vi "rsidr_core_global.vi"() -> ()   [LabVIEW 2020, in "Rohde&Schwarz CMWXP NR FR1 Measurement.lvlib"] (continued)
i9, i10, i11, i12, i13, i14, i15, i16, i17, i18, i19, i20, i21, i22, i23, i24, i25, i26, i27, i28, i29, i30, i31, i32\r\n\nRemote-control command(s):\nCONFigure:NRSub:MEAS<i>:MEValuation:LIMit:QPSK:FERRor"}, {"Level"=5, "Class Only"=FALSE, "Identifier"="RSCMWXPNRFR1M_ATTR_MULTI_EVAL_MEAS_LIMIT_QPSK_IQ_OFFSET", "Descriptive Name"="Multi Eval Meas Limit QPSK IQ Offset", "Data Type"=enum."RawString", "Command"="CONF:NRS:MEAS{instance}:MEV:LIM:QPSK:IQOF", "Access"=enum."Read/Write", "Range Table"="", "Read Callback"="", "Write Callback"="", "Range Callback"="", "Check Callback"="", "Rngtable Callback"="", "Coerce Callback"="", "Supported Models"="", "Instrument Options"="", "Check Status Callback"="", "Flags"=0, "Help"="Defines upper limits for the I/Q origin offset (QPSK modulation). Four different I/Q origin offset limits can be set for four TX power ranges.\n\nSyntax:\nCONFigure:NRSub:MEAS<i>:MEValuation:LIMit:QPSK:IQOFfset <Enable>, <Offset0>, <Offset1>,<Offset2>,<Offset3>\n\n<Enable>\nValid Values:\nOFF: disables the limit check\nON: enables the limit check\n\n<Offset0>\nI/Q origin offset limit for TX power > 10 dBm\nnumeric\nValid Values: -256 dBc to 256 dBc\n\n<Offset1>\nI/Q origin offset limit for TX power > 0 dBm\nnumeric\nValid Values: -256 dBc to 256 dBc\n\n<Offset2>\nI/Q origin offset limit for TX power > -30 dBm\nnumeric\nValid Values: -256 dBc to 256 dBc\n\n<Offset3>\nI/Q origin offset limit for TX power > -40 dBm\nnumeric\nValid Values: -256 dBc to 256 dBc\n\nAvailable Repeated Capabilities:\ninstance: i0, i1, i2, i3, i4, i5, i6, i7, i8, i9, i10, i11, i12, i13, i14, i15, i16, i17, i18, i19, i20, i21, i22, i23, i24, i25, i26, i27, i28, i29, i30, i31, i32\r\n\nRemote-control command(s):\nCONFigure:NRSub:MEAS<i>:MEValuation:LIMit:QPSK:IQOFfset"}, {"Level"=5, "Class Only"=FALSE, "Identifier"="RSCMWXPNRFR1M_ATTR_MULTI_EVAL_MEAS_LIMIT_QPSK_INBAND_EMISSION", "Descriptive Name"="Multi Eval Meas Limit QPSK Inband Emission", "Data Type"=enum."RawString", "Command"="CONF:NRS:MEAS{instance}:MEV:LIM:QPSK:IBE", "Access"=enum."Read/Write", "Range Table"="", "Read Callback"="", "Write Callback"="", "Range Callback"="", "Check Callback"="", "Rngtable Callback"="", "Coerce Callback"="", "Supported Models"="", "Instrument Options"="", "Check Status Callback"="", "Flags"=0, "Help"="Defines parameters used for calculation of an upper limit for the inband emission (QPSK modulation), see 'Inband Emissions Limits'.\n\nSyntax:\nCONFigure:NRSub:MEAS<i>:MEValuation:LIMit:QPSK:IBE <Enable>, <Minimum>, <EVM>, <RBPower>, <IQImageLesser>, <IQImageGreater>\n\n<Enable>\nValid Values:\nOFF: disables the limit check\nON: enables the limit check\n\n<Minimum>\nnumeric\nValid Values: -256 dB to 256 dB\n\n<EVM>\nnumeric\nValid Values: 0 % to 100 %\n\n<RBPower>\nnumeric\nValid Values: -256 dBm to 256 dBm\n\n<IQImageLesser>\nIQ image for low TX power range\nnumeric\nValid Values: -256 dB to 256 dB\n \n<IQImageGreater>\nIQ image for high TX power range\nnumeric\nValid Values: -256 dB  to  256 dB\n\nAvailable Repeated Capabilities:\ninstance: i0, i1, i2, i3, i4, i5, i6, i7, i8, i9, i10, i11, i12, i13, i14, i15, i16, i17, i18, i19, i20, i21, i22, i23, i24, i25, i26, i27, i28, i29, i30, i31, i32\r\n\nRemote-control command(s):\nCONFigure:NRSub:MEAS<i>:MEValuation:LIMit:QPSK:IBE"}, {"Level"=5, "Class Only"=FALSE, "Identifier"="RSCMWXPNRFR1M_ATTR_MULTI_EVAL_MEAS_LIMIT_QPSK_INBAND_EMISSION_IQ_OFFSET", "Descriptive Name"="Multi Eval Meas Limit QPSK Inband Emission IQ Offset", "Data Type"=enum."RawString", "Command"="CONF:NRS:MEAS{instance}:MEV:LIM:QPSK:IBE:IQOF", "Access"=enum."Read/Write", "Range Table"="", "Read Callback"="", "Write Callback"="", "Range Callback"="", "Check Callback"="", "Rngtable Callback"="", "Coerce Callback"="", "Supported Models"="", "Instrument Options"="", "Check Status Callback"="", "Flags"=0, "Help"="Defines I/Q origin offset values used for calculation of an upper limit for the inband emission, for QPSK modulation. Four different values can be set for four TX power ranges.\n\nSyntax:\nCONFigure:NRSub:MEAS<i>:MEValuation:LIMit:QPSK:IBE:IQOFfset <Offset0>, <Offset1>,<Offset2>,<Offset3>\n\n<Offset0>\nI/Q origin offset limit for TX power > 10 dBm\nnumeric\nValid Values: -256 dBc to 256 dBc\n\n<Offset1>\nI/Q origin offset limit for TX power > 0 dBm\nnumeric\nValid Values: -256 dBc to 256 dBc\n\n<Offset2>\nI/Q origin offset limit for TX power > -30 dBm\nnumeric\nValid Values: -256 dBc to 256 dBc\n\n<Offset3>\nI/Q origin offset limit for TX power > -40 dBm\nnumeric\nValid Values: -256 dBc to 256 dBc\n\nAvailable Repeated Capabilities:\ninstance: i0, i1, i2, i3, i4, i5, i6, i7, i8, i9, i10, i11, i12, i13, i14, i15, i16, i17, i18, i19, i20, i21, i22, i23, i24, i25, i26, i27, i28, i29, i30, i31, i32\r\n\nRemote-control command(s):\nCONFigure:NRSub:MEAS<i>:MEValuation:LIMit:QPSK:IBE:IQOFfset"}, {"Level"=5, "Class Only"=FALSE, "Identifier"="RSCMWXPNRFR1M_ATTR_MULTI_EVAL_MEAS_LIMIT_QPSK_EQUALIZER_SPECTRUM_FLATNESS", "Descriptive Name"="Multi Eval Meas Limit QPSK Equalizer Spectrum Flatness", "Data Type"=enum."RawString", "Command"="CONF:NRS:MEAS{instance}:MEV:LIM:QPSK:ESFL", "Access"=enum."Read/Write", "Range Table"="", "Read Callback"="", "Write Callback"="", "Range Callback"="", "Check Callback"="", "Rngtable Callback"="", "Coerce Callback"="", "Supported Models"="", "Instrument Options"="", "Check Status Callback"="", "Flags"=0, "Help"="Defines limits for the equalizer spectrum flatness (QPSK modulation).\n\nSyntax:\nCONFigure:NRSub:MEAS<i>:MEValuation:LIMit:QPSK:ESFLatness <Enable>, <Range1>, <Range2>, <Max1Min2>, <Max2Min1>, <EdgeFrequency>\n\n<Enable>\nValid Values:\nOFF: disables the limit check\nON: enables the limit check\n\n<Range1>\nUpper limit for max(range 1) - min(range 1)\nnumeric\nValid Values: -256 dBpp to 256 dBpp \n\n<Range2>\nUpper limit for max(range 2) - min(range 2)\nnumeric\nValid Values: -256 dBpp to 256 dBpp \n\n<Max1Min2>\nUpper limit for max(range 1) - min(range 2)\nnumeric\nValid Values: -256 dB to 256 dB \n\n<Max2Min1>\nUpper limit for max(range 2) - min(range 1)\nnumeric\nValid Values: -256 dB to 256 dB\n\n<EdgeFrequency>\nBand edge distance of border between range 1 and range 2\nValid Values:\n0 MHz to 20 MHz\n\nAvailable Repeated Capabilities:\ninstance: i0, i1, i2, i3, i4, i5, i6, i7, i8, i9, i10, i11, i12, i13, i14, i15, i16, i17, i18, i19, i20, i21, i22, i23, i24, i25, i26, i27, i28, i29, i30, i31, i32\r\n\nRemote-control command(s):\nCONFigure:NRSub:MEAS<i>:MEValuation:LIMit:QPSK:ESFLatness"}, {"Level"=4, "Class Only"=TRUE, "Identifier"="", "Descriptive Name"="QAM", "Data Type"=enum."ViInt32", "Command"="", "Access"=enum."Read Only", "Range Table"="", "Read Callback"="", "Write Callback"="", "Range Callback"="", "Check Callback"="", "Rngtable Callback"="", "Coerce Callback"="", "Supported Models"="", "Instrument Options"="", "Check Status Callback"="", "Flags"=0, "Help"="16-QAM / 64-QAM / 256-QAM modulation  limits definition."}, {"Level"=5, "Class Only"=FALSE, "Identifier"="RSCMWXPNRFR1M_ATTR_MULTI_EVAL_MEAS_LIMIT_QAM_EVM", "Descriptive Name"="Multi Eval Meas Limit QAM EVM", "Data Type"=enum."RawString", "Command"="CONF:NRS:MEAS{instance}:MEV:LIM:QAM{QAM}:EVM", "Access"=enum."Read/Write", "Range Table"="", "Read Callback"="", "Write Callback"="", "Range Callback"="", "Check Callback"="", "Rngtable Callback"="", "Coerce Callback"="", "Supported Models"="", "Instrument Options"="", "Check Status Callback"="", "Flags"=0, "Help"="Defines upper limits for the RMS and peak values of the error vector magnitude (EVM) for QAM modulations.\n\nSyntax:\nCONFigure:NRSub:MEAS<i>:MEValuation:LIMit:QAM<order>:EVMagnitude <RMS>, <Peak>\n\n<RMS>\nnumeric | ON | OFF\nValid Values:\n0 % to 100 %\n  \n<Peak>\nnumeric | ON | OFF\nValid Values:\n0 % to 100 %\n\nAvailable Repeated Capabilities:\ninstance: i0, i1, i2, i3, i4, i5, i6, i7, i8, i9, i10, i11, i12, i13, i14, i15, i16, i17, i18, i19, i20, i21, i22, i23, i24, i25, i26, i27, i28, i29, i30, i31, i32\r\nQAM: QAM16, QAM64, QAM256\r\n\nRemote-control command(s):\nCONFigure:NRSub:MEAS<i>:MEValuation:LIMit:QAM<order>:EVMagnitude"}, {"Level"=5, "Class Only"=FALSE, "Identifier"="RSCMWXPNRFR1M_ATTR_MULTI_EVAL_MEAS_LIMIT_QAM_MERR", "Descriptive Name"="Multi Eval Meas Limit QAM MERR", "Data Type"=enum."RawString", "Command"="CONF:NRS:MEAS{instance}:MEV:LIM:QAM{QAM}:MERR", "Access"=enum."Read/Write", "Range Table"="", "Read Callback"="", "Write Callback"="", "Range Callback"="", "Check Callback"="", "Rngtable Callback"="", "Coerce Callback"="", "Supported Models"="", "Instrument Options"="", "Check Status Callback"="", "Flags"=0, "Help"="Defines upper limits for the RMS and peak values of the magnitude error for QAM modulations.\n\nSyntax:\nCONFigure:NRSub:MEAS<i>:MEValuation:LIMit:QAM<order>:MERRor <RMS>, <Peak>\n\n<RMS>\nnumeric | ON | OFF\nValid Values:\n0 % to 100 %\n  \n<Peak>\nnumeric | ON | OFF\nValid Values:\n0 % to 100 %\n\nAvailable Repeated Capabilities:\ninstance: i0, i1, i2, i3, i4, i5, i6, i7, i8, i9, i10, i11, i12, i13, i14, i15, i16, i17, i18, i19, i20, i21, i22, i23, i24, i25, i26, i27, i28, i29, i30, i31, i32\r\nQAM: QAM16, QAM64, QAM256\r\n\nRemote-control command(s):\nCONFigure:NRSub:MEAS<i>:MEValuation:LIMit:QAM<order>:MERRor"}, {"Level"=5, "Class Only"=FALSE, "Identifier"="RSCMWXPNRFR1M_ATTR_MULTI_EVAL_MEAS_LIMIT_QAM_PERR", "Descriptive Name"="Multi Eval Meas Limit QAM PERR", "Data Type"=enum."RawString", "Command"="CONF:NRS:MEAS{instance}:MEV:LIM:QAM{QAM}:PERR", "Access"=enum."Read/Write", "Range Table"="", "Read Callback"="", "Write Callback"="", "Range Callback"="", "Check Callback"="", "Rngtable Callback"="", "Coerce Callback"="", "Supported Models"="", "Instrument Options"="", "Check Status Callback"="", "Flags"=0, "Help"="Defines symmetric limits for the RMS and peak values of the phase error for QAM modulations. The limit check fails if the absolute value of the measured phase error exceeds the specified values.\n\nSyntax:\nCONFigure:NRSub:MEAS<i>:MEValuation:LIMit:QAM<order>:PERRor <RMS>, <Peak>\n\n<RMS>\nnumeric | ON | OFF\nValid Values:\n0 % to 100 %\n  \n<Peak>\nnumeric | ON | OFF\nValid Values:\n0 % to 100 %\n\nAvailable Repeated Capabilities:\ninstance: i0, i1, i2, i3, i4, i5, i6, i7, i8, i9, i10, i11, i12, i13, i14, i15, i16, i17, i18, i19, i20, i21, i22, i23, i24, i25, i26, i27, i28, i29, i30, i31, i32\r\nQAM: QAM16, QAM64, QAM256\r\n\nRemote-control command(s):\nCONFigure:NRSub:MEAS<i>:MEValuation:LIMit:QAM<order>:PERRor"}, {"Level"=5, "Class Only"=FALSE, "Identifier"="RSCMWXPNRFR1M_ATTR_MULTI_EVAL_MEAS_LIMIT_QAM_FERR_ENABLED", "Descriptive Name"="Multi Eval Meas Limit QAM FERR Enabled", "Data Type"=enum."ViBoolean", "Command"="CONF:NRS:MEAS{instance}:MEV:LIM:QAM{QAM}:FERR", "Access"=enum."Read/Write", "Range Table"="", "Read Callback"="", "Write Callback"="", "Range Callback"="", "Check Callback"="", "Rngtable Callback"="", "Coerce Callback"="", "Supported Models"="", "Instrument Options"="", "Check Status Callback"="", "Flags"=0, "Help"="Defines an upper limit for the carrier frequency error (QAM modulations).\n\nAvailable Repeated Capabilities:\ninstance: i0, i1, i2, i3, i4, i5, i6, i7, i8, i9, i10, i11, i12, i13, i14, i15, i16, i17, i18, i19, i20, i21, i22, i23, i24, i25, i26, i27, i28, i29, i30, i31, i32\r\nQAM: QAM16, QAM64, QAM256\r\n\nRemote-control command(s):\nCONFigure:NRSub:MEAS<i>:MEValuation:LIMit:QAM<order>:FERRor"}, {"Level"=5, "Class Only"=FALSE, "Identifier"="RSCMWXPNRFR1M_ATTR_MULTI_EVAL_MEAS_LIMIT_QAM_FERR", "Descriptive Name"="Multi Eval Meas Limit QAM FERR", "Data Type"=enum."ViReal64", "Command"="CONF:NRS:MEAS{instance}:MEV:LIM:QAM{QAM}:FERR", "Access"=enum."Read/Write", "Range Table"="rsCmwxpNrFr1M_rngFERR", "Read Callback"="", "Write Callback"="", "Range Callback"="", "Check Callback"="", "Rngtable Callback"="", "Coerce Callback"="", "Supported Models"="", "Instrument Options"="", "Check Status Callback"="", "Flags"=0, "Help"="Defines an upper limit for the carrier frequency error (QAM modulations).\n\nAvailable Repeated Capabilities:\ninstance: i0, i1, i2, i3, i4, i5, i6, i7, i8, i9, i10, i11, i12, i13, i14, i15, i16, i17, i18, i19, i20, i21, i22, i23, i24, i25, i26, i27, i28, i29, i30, i31, i32\r\nQAM: QAM16, QAM64, QAM256\r\n\nRemote-control command(s):\nCONFigure:NRSub:MEAS<i>:MEValuation:LIMit:QAM<order>:FERRor"}, {"Level"=5, "Class Only"=FALSE, "Identifier"="RSCMWXPNRFR1M_ATTR_MULTI_EVAL_MEAS_LIMIT_QAM_IQ_OFFSET", "Descriptive Name"="Multi Eval Meas Limit QAM IQ Offset", "Data Type"=enum."RawString", "Command"="CONF:NRS:MEAS{instance}:MEV:LIM:QAM{QAM}:IQOF", "Access"=enum."Read/Write", "Range Table"="", "Read Callback"="", "Write Callback"="", "Range Callback"="", "Check Callback"="", "Rngtable Callback"="", "Coerce Callback"="", "Supported Models"="", "Instrument Options"="", "Check Status Callback"="", "Flags"=0, "Help"="Defines upper limits for the I/Q origin offset (QAM modulations). Four different I/Q origin offset limits can be set for four TX power ranges.\n\nSyntax:\nCONFigure:NRSub:MEAS<i>:MEValuation:LIMit:QAM<order>:IQOFfset <Enable>, <Offset0>, <Offset1>,<Offset2>,<Offset3>\n\n<Enable>\nValid Values:\nOFF: disables the limit check\nON: enables the limit check\n\n<Offset0>\nI/Q origin offset limit for TX power > 10 dBm\nnumeric\nValid Values: -256 dBc to 256 dBc\n\n<Offset1>\nI/Q origin offset limit for TX power > 0 dBm\nnumeric\nValid Values: -256 dBc to 256 dBc\n\n<Offset2>\nI/Q origin offset limit for TX power > -30 dBm\nnumeric\nValid Values: -256 dBc to 256 dBc\n\n<Offset3>\nI/Q origin offset limit for TX power > -40 dBm\nnumeric\nValid Values: -256 dBc to 256 dBc\n\nAvailable Repeated Capabilities:\ninstance: i0, i1, i2, i3, i4, i5, i6, i7, i8, i9, i10, i11, i12, i13, i14, i15, i16, i17, i18, i19, i20, i21, i22, i23, i24, i25, i26, i27, i28, i29, i30, i31, i32\r\nQAM: QAM16, QAM64, QAM256\r\n\nRemote-control command(s):\nCONFigure:NRSub:MEAS<i>:MEValuation:LIMit:QAM<order>:IQOFfset"}, {"Level"=5, "Class Only"=FALSE, "Identifier"="RSCMWXPNRFR1M_ATTR_MULTI_EVAL_MEAS_LIMIT_QAM_INBAND_EMISSION", "Descriptive Name"="Multi Eval Meas Limit QAM Inband Emission", "Data Type"=enum."RawString", "Command"="CONF:NRS:MEAS{instance}:MEV:LIM:QAM{QAM}:IBE", "Access"=enum."Read/Write", "Range Table"="", "Read Callback"="", "Write Callback"="", "Range Callback"="", "Check Callback"="", "Rngtable Callback"="", "Coerce Callback"="", "Supported Models"="", "Instrument Options"="", "Check Status Callback"="", "Flags"=0, "Help"="Defines parameters used for calculation of an upper limit for the inband emission (QAM modulations), see 'Inband Emissions Limits'.\n\nSyntax:\nCONFigure:NRSub:MEAS<i>:MEValuation:LIMit:QAM<order>:IBE <Enable>, <Minimum>, <EVM>, <RBPower>, <IQImageLesser>, <IQImageGreater>\n\n<Enable>\nValid Values:\nOFF: disables the limit check\nON: enables the limit check\n\n<Minimum>\nnumeric\nValid Values: -256 dB to 256 dB\n\n<EVM>\nnumeric\nValid Values: 0 % to 100 %\n\n<RBPower>\nnumeric\nValid Values: -256 dBm to 256 dBm\n\n<IQImageLesser>\nIQ image for low TX power range\nnumeric\nValid Values: -256 dB to 256 dB\n \n<IQImageGreater>\nIQ image for high TX power range\nnumeric\nValid Values: -256 dB  to  256 dB\n\nAvailable Repeated Capabilities:\ninstance: i0, i1, i2, i3, i4, i5, i6, i7, i8, i9, i10, i11, i12, i13, i14, i15, i16, i17, i18, i19, i20, i21, i22, i23, i24, i25, i26, i27, i28, i29, i30, i31, i32\r\nQAM: QAM16, QAM64, QAM256\r\n\nRemote-control command(s):\nCONFigure:NRSub:MEAS<i>:MEValuation:LIMit:QAM<order>:IBE"}, {"Level"=5, "Class Only"=FALSE, "Identifier"="RSCMWXPNRFR1M_ATTR_MULTI_EVAL_MEAS_LIMIT_QAM_INBAND_EMISSION_IQ_OFFSET", "Descriptive Name"="Multi Eval Meas Limit QAM Inband Emission IQ Offset", "Data Type"=enum."RawString", "Command"="CONF:NRS:MEAS{instance}:MEV:LIM:QAM{QAM}:IBE:IQOF", "Access"=enum."Read/Write", "Range Table"="", "Read Callback"="", "Write Callback"="", "Range Callback"="", "Check Callback"="", "Rngtable Callback"="", "Coerce Callback"="", "Supported Models"="", "Instrument Options"="", "Check Status Callback"="", "Flags"=0, "Help"="Defines I/Q origin offset values used for calculation of an upper limit for the inband emission, for QAM modulations. Four different values can be set for four TX power ranges.\n\nSyntax:\nCONFigure:NRSub:MEAS<i>:MEValuation:LIMit:QAM<order>:IBE:IQOFfset <Offset0>, <Offset1>,<Offset2>,<Offset3>\n\n<Offset0>\nI/Q origin offset limit for TX power > 10 dBm\nnumeric\nValid Values: -256 dBc to 256 dBc\n\n<Offset1>\nI/Q origin offset limit for TX power > 0 dBm\nnumeric\nValid Values: -256 dBc to 256 dBc\n\n<Offset2>\nI/Q origin offset limit for TX power > -30 dBm\nnumeric\nValid Values: -256 dBc to 256 dBc\n\n<Offset3>\nI/Q origin offset limit for TX power > -40 dBm\nnumeric\nValid Values: -256 dBc to 256 dBc\n\nAvailable Repeated Capabilities:\ninstance: i0, i1, i2, i3, i4, i5, i6, i7, i8, i9, i10, i11, i12, i13, i14, i15, i16, i17, i18, i19, i20, i21, i22, i23, i24, i25, i26, i27, i28, i29, i30, i31, i32\r\nQAM: QAM16, QAM64, QAM256\r\n\nRemote-control command(s):\nCONFigure:NRSub:MEAS<i>:MEValuation:LIMit:QAM<order>:IBE:IQOFfset"}, {"Level"=5, "Class Only"=FALSE, "Identifier"="RSCMWXPNRFR1M_ATTR_MULTI_EVAL_MEAS_LIMIT_QAM_EQUALIZER_SPECTRUM_FLATNESS", "Descriptive Name"="Multi Eval Meas Limit QAM Equalizer Spectrum Flatness", "Data Type"=enum."RawString", "Command"="CONF:NRS:MEAS{instance}:MEV:LIM:QAM{QAM}:ESFL", "Access"=enum."Read/Write", "Range Table"="", "Read Callback"="", "Write Callback"="", "Range Callback"="", "Check Callback"="", "Rngtable Callback"="", "Coerce Callback"="", "Supported Models"="", "Instrument Options"="", "Check Status Callback"="", "Flags"=0, "Help"="Defines limits for the equalizer spectrum flatness (QAM modulations).\n\nSyntax:\nCONFigure:NRSub:MEAS<i>:MEValuation:LIMit:QAM<order>:ESFLatness <Enable>, <Range1>, <Range2>, <Max1Min2>, <Max2Min1>, <EdgeFrequency>\n\n<Enable>\nValid Values:\nOFF: disables the limit check\nON: enables the limit check\n\n<Range1>\nUpper limit for max(range 1) - min(range 1)\nnumeric\nValid Values: -256 dBpp to 256 dBpp \n\n<Range2>\nUpper limit for max(range 2) - min(range 2)\nnumeric\nValid Values: -256 dBpp to 256 dBpp \n\n<Max1Min2>\nUpper limit for max(range 1) - min(range 2)\nnumeric\nValid Values: -256 dB to 256 dB \n\n<Max2Min1>\nUpper limit for max(range 2) - min(range 1)\nnumeric\nValid Values: -256 dB to 256 dB\n\n<EdgeFrequency>\nBand edge distance of border between range 1 and range 2\nValid Values:\n0 MHz to 20 MHz\n\nAvailable Repeated Capabilities:\ninstance: i0, i1, i2, i3, i4, i5, i6, i7, i8, i9, i10, i11, i12, i13, i14, i15, i16, i17, i18, i19, i20, i21, i22, i23, i24, i25, i26, i27, i28, i29, i30, i31, i32\r\nQAM: QAM16, QAM64, QAM256\r\n\nRemote-control command(s):\nCONFigure:NRSub:MEAS<i>:MEValuation:LIMit:QAM<order>:ESFLatness"}, {"Level"=3, "Class Only"=TRUE, "Identifier"="", "Descriptive Name"="Spectrum", "Data Type"=enum."ViInt32", "Command"="", "Access"=enum."Read Only", "Range Table"="", "Read Callback"="", "Write Callback"="", "Range Callback"="", "Check Callback"="", "Rngtable Callback"="", "Coerce Callback"="", "Supported Models"="", "Instrument Options"="", "Check Status Callback"="", "Flags"=0, "Help"="Spectrum limits definition."}, {"Level"=4, "Class Only"=FALSE, "Identifier"="RSCMWXPNRFR1M_ATTR_MULTI_EVAL_MEAS_LIMIT_OBW_ENABLED", "Descriptive Name"="Multi Eval Meas Limit OBW Enabled", "Data Type"=enum."ViBoolean", "Command"="CONF:NRS:MEAS{instance}:MEV:LIM:SEM:OBWL:CBAN{Bandwidth}", "Access"=enum."Read/Write", "Range Table"="", "Read Callback"="", "Write Callback"="", "Range Callback"="", "Check Callback"="", "Rngtable Callback"="", "Coerce Callback"="", "Supported Models"="", "Instrument Options"="", "Check Status Callback"="", "Flags"=0, "Help"="Defines an upper limit for the occupied bandwidth, depending on the channel bandwidth (for NR SA).\n\nAvailable Repeated Capabilities:\ninstance: i0, i1, i2, i3, i4, i5, i6, i7, i8, i9, i10, i11, i12, i13, i14, i15, i16, i17, i18, i19, i20, i21, i22, i23, i24, i25, i26, i27, i28, i29, i30, i31, i32\r\nBandwidth: bw5, bw10, bw15, bw20, bw25, bw30, bw40, bw50, bw60, bw80, bw90, bw100\r\n\nRemote-control command(s):\nCONFigure:NRSub:MEAS<i>:MEValuation:LIMit:SEMask:OBWLimit:CBANdwidth<bw>"}, {"Level"=4, "Class Only"=FALSE, "Identifier"="RSCMWXPNRFR1M_ATTR_MULTI_EVAL_MEAS_LIMIT_OBW", "Descriptive Name"="Multi Eval Meas Limit OBW", "Data Type"=enum."ViReal64", "Command"="CONF:NRS:MEAS{instance}:MEV:LIM:SEM:OBWL:CBAN{Bandwidth}", "Access"=enum."Read/Write", "Range Table"="rsCmwxpNrFr1M_rngLimitOBW", "Read Callback"="", "Write Callback"="", "Range Callback"="", "Check Callback"="", "Rngtable Callback"="", "Coerce Callback"="", "Supported Models"="", "Instrument Options"="", "Check Status Callback"="", "Flags"=0, "Help"="Defines an upper limit for the occupied bandwidth, depending on the channel bandwidth (for NR SA).\n\nAvailable Repeated Capabilities:\ninstance: i0, i1, i2, i3, i4, i5, i6, i7, i8, i9, i10, i11, i12, i13, i14, i15, i16, i17, i18, i19, i20, i21, i22, i23, i24, i25, i26, i27, i28, i29, i30, i31, i32\r\nBandwidth: bw5, bw10, bw15, bw20, bw25, bw30, bw40, bw50, bw60, bw80, bw90, bw100\r\n\nRemote-control command(s):\nCONFigure:NRSub:MEAS<i>:MEValuation:LIMit:SEMask:OBWLimit:CBANdwidth<bw>"}, {"Level"=4, "Class Only"=FALSE, "Identifier"="RSCMWXPNRFR1M_ATTR_MULTI_EVAL_MEAS_LIMIT_EMISSION_MASK", "Descriptive Name"="Multi Eval Meas Limit Emission Mask", "Data Type"=enum."RawString", "Command"="CONF:NRS:MEAS{instance}:MEV:LIM:SEM:AREA{Area}:CBAN{Bandwidth}", "Access"=enum."Read/Write", "Range Table"="", "Read Callback"="", "Write Callback"="", "Range Callback"="", "Check Callback"="", "Rngtable Callback"="", "Coerce Callback"="", "Supported Models"="", "Instrument Options"="", "Check Status Callback"="", "Flags"=0, "Help"="Defines general requirements for the emission mask area number <area> (for NR SA). The activation state, the area borders, an upper limit and the resolution bandwidth must be specified.\nThe emission mask applies to the channel bandwidth <bw>.\n\nSyntax:\nCONFigure:NRSub:MEAS<i>:MEValuation:LIMit:SEMask:AREA<area>:CBANdwidth<bw> <Enable>, <FrequencyStart>, <FrequencyEnd>, <Level>, <RBW>\n\n<bw>\nChannel bandwidth in MHz\nValid Values: 50, 100, 200, 400\n \n<area>\nNumber of the emission mask area\nValid Values: 1 to 12\n\n<Enable>\nValid Values:\nOFF: disables the check of these requirements\nON: enables the check of these requirements\n \n<FrequencyStart>\nStart frequency of the area, relative to the edges of the channel bandwidth\nnumeric\nValid Values: 0 MHz to 405 MHz (less, depending on <bw>) \n \n<FrequencyEnd>\nStop frequency of the area, relative to the edges of the channel bandwidth\nnumeric\nValid Values: 0 MHz to 405 MHz (less, depending on <bw>)\n\n<Level>\nUpper limit for the area\nnumeric\nValid Values: -256 dBm to 256 dBm\n\n<RBW>\nResolution bandwidth to be used for the area (1 MHz)\nValid Values: M1\n\nAvailable Repeated Capabilities:\ninstance: i0, i1, i2, i3, i4, i5, i6, i7, i8, i9, i10, i11, i12, i13, i14, i15, i16, i17, i18, i19, i20, i21, i22, i23, i24, i25, i26, i27, i28, i29, i30, i31, i32\r\nArea: a1, a2, a3, a4, a5, a6, a7, a8, a9, a10, a11, a12\r\nBandwidth: bw5, bw10, bw15, bw20, bw25, bw30, bw40, bw50, bw60, bw80, bw90, bw100\r\n\nRemote-control command(s):\nCONFigure:NRSub:MEAS<i>:MEValuation:LIMit:SEMask:AREA<area>:CBANdwidth<bw>"}, {"Level"=4, "Class Only"=FALSE, "Identifier"="RSCMWXPNRFR1M_ATTR_MULTI_EVAL_MEAS_LIMIT_ACLR_ENABLED", "Descriptive Name"="Multi Eval Meas Limit ACLR Enabled", "Data Type"=enum."RawString", "Command"="CONF:NRS:MEAS{instance}:MEV:LIM:ACLR:NR:CBAN{Bandwidth}", "Access"=enum."Read/Write", "Range Table"="", "Read Callback"="", "Write Callback"="", "Range Callback"="", "Check Callback"="", "Rngtable Callback"="", "Coerce Callback"="", "Supported Models"="", "Instrument Options"="", "Check Status Callback"="", "Flags"=0, "Help"="Defines relative and absolute limits for the ACLR measured in an adjacent NR channel (for NR SA). The settings are defined separately for each channel bandwidth.\n\nSyntax:\nCONFigure:NRSub:MEAS<i>:MEValuation:LIMit:ACLR:NR:CBANdwidth<bw> <RelativeLevel>, <AbsoluteLevel>\n\n<bw>\nChannel bandwidth in MHz\nValid Values: 50, 100, 200, 400\n \n<RelativeLevel>\nRelative lower ACLR limit without test tolerance\nON | OFF\n\n<AbsoluteLevel>\nON | OFF\nON | OFF enables or disables the limit check.\n\nAvailable Repeated Capabilities:\ninstance: i0, i1, i2, i3, i4, i5, i6, i7, i8, i9, i10, i11, i12, i13, i14, i15, i16, i17, i18, i19, i20, i21, i22, i23, i24, i25, i26, i27, i28, i29, i30, i31, i32\r\nBandwidth: bw5, bw10, bw15, bw20, bw25, bw30, bw40, bw50, bw60, bw80, bw90, bw100\r\n\nRemote-control command(s):\nCONFigure:NRSub:MEAS<i>:MEValuation:LIMit:ACLR:NR:CBANdwidth<bw>"}, {"Level"=4, "Class Only"=FALSE, "Identifier"="RSCMWXPNRFR1M_ATTR_MULTI_EVAL_MEAS_LIMIT_ACLR", "Descriptive Name"="Multi Eval Meas Limit ACLR", "Data Type"=enum."RawString", "Command"="CONF:NRS:MEAS{instance}:MEV:LIM:ACLR:NR:CBAN{Bandwidth}", "Access"=enum."Read/Write", "Range Table"="", "Read Callback"="", "Write Callback"="", "Range Callback"="", "Check Callback"="", "Rngtable Callback"="", "Coerce Callback"="", "Supported Models"="", "Instrument Options"="", "Check Status Callback"="", "Flags"=0, "Help"="Defines relative and absolute limits for the ACLR measured in an adjacent NR channel (for NR SA). The settings are defined separately for each channel bandwidth.\n\nSyntax:\nCONFigure:NRSub:MEAS<i>:MEValuation:LIMit:ACLR:NR:CBANdwidth<bw> <RelativeLevel>, <AbsoluteLevel>\n\n<bw>\nChannel bandwidth in MHz\nValid Values: 50, 100, 200, 400\n \n<RelativeLevel>\nRelative lower ACLR limit without test tolerance\nnumeric\nValid Values: -256 dB to 256 dB\n\n<AbsoluteLevel>\n numeric\nValid Values: -256 dBm to 256 dBm\n\nAvailable Repeated Capabilities:\ninstance: i0, i1, i2, i3, i4, i5, i6, i7, i8, i9, i10, i11, i12, i13, i14, i15, i16, i17, i18, i19, i20, i21, i22, i23, i24, i25, i26, i27, i28, i29, i30, i31, i32\r\nBandwidth: bw5, bw10, bw15, bw20, bw25, bw30, bw40, bw50, bw60, bw80, bw90, bw100\r\n\nRemote-control command(s):\nCONFigure:NRSub:MEAS<i>:MEValuation:LIMit:ACLR:NR:CBANdwidth<bw>"}, {"Level"=4, "Class Only"=FALSE, "Identifier"="RSCMWXPNRFR1M_ATTR_MULTI_EVAL_MEAS_LIMIT_ACLR_TEST_TOLERANCE", "Descriptive Name"="Multi Eval Meas Limit ACLR Test Tolerance", "Data Type"=enum."RawString", "Command"="CONF:NRS:MEAS{instance}:MEV:LIM:ACLR:TTOL", "Access"=enum."Read/Write", "Range Table"="", "Read Callback"="", "Write Callback"="", "Range Callback"="", "Check Callback"="", "Rngtable Callback"="", "Coerce Callback"="", "Supported Models"="", "Instrument Options"="", "Check Status Callback"="", "Flags"=0, "Help"="Defines the test tolerance for relative ACLR limits, depending on the carrier frequency.\n\nSyntax:\nCONFigure:NRSub:MEAS<i>:MEValuation:LIMit:ACLR:TTOLerance <TestTolSub4GHz>, <TestTolSub6GHz>\n\n<TestTolSub4GHz>\nTest tolerance for carrier frequencies  4 GHz\nValid Values:\n-3 dB to 3 dB\n\n<TestTolSub6GHz>\nTest tolerance for carrier frequencies > 4 GHz\nValid Values:\n-3 dB to 3 dB\n\nAvailable Repeated Capabilities:\ninstance: i0, i1, i2, i3, i4, i5, i6, i7, i8, i9, i10, i11, i12, i13, i14, i15, i16, i17, i18, i19, i20, i21, i22, i23, i24, i25, i26, i27, i28, i29, i30, i31, i32\r\n\nRemote-control command(s):\nCONFigure:NRSub:MEAS<i>:MEValuation:LIMit:ACLR:TTOLerance"}, {"Level"=4, "Class Only"=FALSE, "Identifier"="RSCMWXPNRFR1M_ATTR_MULTI_EVAL_MEAS_LIMIT_ACLR_EN_DC_ENABLED", "Descriptive Name"="Multi Eval Meas Limit ACLR EN-DC Enabled", "Data Type"=enum."ViBoolean", "Command"="CONF:NRS:MEAS{instance}:MEV:LIM:ACLR:ENDC", "Access"=enum."Read/Write", "Range Table"="", "Read Callback"="", "Write Callback"="", "Range Callback"="", "Check Callback"="", "Rngtable Callback"="", "Coerce Callback"="", "Supported Models"="", "Instrument Options"="", "Check Status Callback"="", "Flags"=0, "Help"="Defines a relative limit for the ACLR measured in an adjacent channel in EN-DC mode.\n\nAvailable Repeated Capabilities:\ninstance: i0, i1, i2, i3, i4, i5, i6, i7, i8, i9, i10, i11, i12, i13, i14, i15, i16, i17, i18, i19, i20, i21, i22, i23, i24, i25, i26, i27, i28, i29, i30, i31, i32\r\n\nRemote-control command(s):\nCONFigure:NRSub:MEAS<i>:MEValuation:LIMit:ACLR:ENDC"}, {"Level"=4, "Class Only"=FALSE, "Identifier"="RSCMWXPNRFR1M_ATTR_MULTI_EVAL_MEAS_LIMIT_ACLR_EN_DC", "Descriptive Name"="Multi Eval Meas Limit ACLR EN-DC", "Data Type"=enum."ViReal64", "Command"="CONF:NRS:MEAS{instance}:MEV:LIM:ACLR:ENDC", "Access"=enum."Read/Write", "Range Table"="rsCmwxpNrFr1M_rngRelativeLevel", "Read Callback"="", "Write Callback"="", "Range Callback"="", "Check Callback"="", "Rngtable Callback"="", "Coerce Callback"="", "Supported Models"="", "Instrument Options"="", "Check Status Callback"="", "Flags"=0, "Help"="Defines a relative limit for the ACLR measured in an adjacent channel in EN-DC mode.\n\nAvailable Repeated Capabilities:\ninstance: i0, i1, i2, i3, i4, i5, i6, i7, i8, i9, i10, i11, i12, i13, i14, i15, i16, i17, i18, i19, i20, i21, i22, i23, i24, i25, i26, i27, i28, i29, i30, i31, i32\r\n\nRemote-control command(s):\nCONFigure:NRSub:MEAS<i>:MEValuation:LIMit:ACLR:ENDC"}, {"Level"=4, "Class Only"=FALSE, "Identifier"="RSCMWXPNRFR1M_ATTR_MULTI_EVAL_MEAS_LIMIT_ACLR_UTRA_CHANNEL_BANDWIDTH", "Descriptive Name"="Multi Eval Meas Limit ACLR UTRA Channel Bandwidth", "Data Type"=enum."RawString", "Command"="CONF:NRS:MEAS{instance}:MEV:LIM:ACLR:UTRA{UTRA}:CBAN{Bandwidth}", "Access"=enum."Read/Write", "Range Table"="", "Read Callback"="", "Write Callback"="", "Range Callback"="", "Check Callback"="", "Rngtable Callback"="", "Coerce Callback"="", "Supported Models"="", "Instrument Options"="", "Check Status Callback"="", "Flags"=0, "Help"="Defines relative and absolute limits for the ACLR measured in the first or second adjacent UTRA channel, depending on UTRA<no> (for NR SA). The settings are defined separately for each channel bandwidth.\n\nCONFigure:NRSub:MEAS<i>:MEValuation:LIMit:ACLR:UTRA<no>:CBANdwidth<bw> <RelativeLevel>, <AbsoluteLevel>\n\n<RelativeLevel> - numeric | ON | OFF\nRelative lower ACLR limit without test tolerance\nValid Values:\n-256 dB to 256 dB\n\n<AbsolutePower> - numeric | ON | OFF\nValid Values:\n-256 dBm to 256 dBm\n\nAvailable Repeated Capabilities:\ninstance: i0, i1, i2, i3, i4, i5, i6, i7, i8, i9, i10, i11, i12, i13, i14, i15, i16, i17, i18, i19, i20, i21, i22, i23, i24, i25, i26, i27, i28, i29, i30, i31, i32\r\nUTRA: UTRA1, UTRA2\r\nBandwidth: bw5, bw10, bw15, bw20, bw25, bw30, bw40, bw50, bw60, bw80, bw90, bw100\r\n\nRemote-control command(s):\nCONFigure:NRSub:MEAS<i>:MEValuation:LIMit:ACLR:UTRA<no>:CBANdwidth<bw>"}, {"Level"=4, "Class Only"=FALSE, "Identifier"="RSCMWXPNRFR1M_ATTR_MULTI_EVAL_MEAS_LIMIT_SEM_OBW_ENABLED", "Descriptive Name"="Multi Eval Meas Limit SEM OBW Enabled", "Data Type"=enum."ViBoolean", "Command"="CONF:NRS:MEAS{instance}:MEV:LIM:SEM:OBWL:ENDC", "Access"=enum."Read/Write", "Range Table"="", "Read Callback"="", "Write Callback"="", "Range Callback"="", "Check Callback"="", "Rngtable Callback"="", "Coerce Callback"="", "Supported Models"="", "Instrument Options"="", "Check Status Callback"="", "Flags"=0, "Help"="Defines an upper limit for the occupied bandwidth, for EN-DC measurements.\n\nAvailable Repeated Capabilities:\ninstance: i0, i1, i2, i3, i4, i5, i6, i7, i8, i9, i10, i11, i12, i13, i14, i15, i16, i17, i18, i19, i20, i21, i22, i23, i24, i25, i26, i27, i28, i29, i30, i31, i32\r\n\nRemote-control command(s):\nCONFigure:NRSub:MEAS<i>:MEValuation:LIMit:SEMask:OBWLimit:ENDC"}, {"Level"=4, "Class Only"=FALSE, "Identifier"="RSCMWXPNRFR1M_ATTR_MULTI_EVAL_MEAS_LIMIT_SEM_TEST_TOLERANCE", "Descriptive Name"="Multi Eval Meas Limit SEM Test Tolerance", "Data Type"=enum."RawString", "Command"="CONF:NRS:MEAS{instance}:MEV:LIM:SEM:TTOL", "Access"=enum."Read/Write", "Range Table"="", "Read Callback"="", "Write Callback"="", "Range Callback"="", "Check Callback"="", "Rngtable Callback"="", "Coerce Callback"="", "Supported Models"="", "Instrument Options"="", "Check Status Callback"="", "Flags"=0, "Help"="Defines the test tolerance for spectrum emission masks, depending on the carrier frequency.\n\nSyntax:\nCONFigure:NRSub:MEAS<i>:MEValuation:LIMit:SEMask:TTOLerance <TestTolSub3GHz>, <TestTolSub4GHz>, <TestTolSub6GHz>\n\n<TestTolSub3GHz>\nTest tolerance for carrier frequencies  3 GHz\nValid Values:\n-3 dB to 3 dB\n\n<TestTolSub4GHz>\nTest tolerance for carrier frequencies > 3 GHz and  4.2 GHz\nValid Values:\n-3 dB to 3 dB\n\n<TestTolSub6GHz>\nTest tolerance for carrier frequencies > 4.2 GHz\nValid Values:\n-3 dB to 3 dB\n\nAvailable Repeated Capabilities:\ninstance: i0, i1, i2, i3, i4, i5, i6, i7, i8, i9, i10, i11, i12, i13, i14, i15, i16, i17, i18, i19, i20, i21, i22, i23, i24, i25, i26, i27, i28, i29, i30, i31, i32\r\n\nRemote-control command(s):\nCONFigure:NRSub:MEAS<i>:MEValuation:LIMit:SEMask:TTOLerance"}, {"Level"=4, "Class Only"=FALSE, "Identifier"="RSCMWXPNRFR1M_ATTR_MULTI_EVAL_MEAS_LIMIT_SEM_EN_DC", "Descriptive Name"="Multi Eval Meas Limit SEM EN-DC", "Data Type"=enum."RawString", "Command"="CONF:NRS:MEAS{instance}:MEV:LIM:SEM:AREA{Area}:ENDC", "Access"=enum."Read/Write", "Range Table"="", "Read Callback"="", "Write Callback"="", "Range Callback"="", "Check Callback"="", "Rngtable Callback"="", "Coerce Callback"="", "Supported Models"="", "Instrument Options"="", "Check Status Callback"="", "Flags"=0, "Help"="Defines general requirements for the emission mask area number <no> (for EN-DC). The activation state, the area borders, an upper limit and the resolution bandwidth must be specified.\n\nSyntax:\nCONFigure:NRSub:MEAS<i>:MEValuation:LIMit:SEMask:AREA<no>:ENDC <Enable>, <FrequencyStart>, <FrequencyEnd>, <Level>, <RBW>\n\n<Enable>\nValid Values:\nOFF\nON\n\n<FrequencyStart>\nStart frequency of the area, relative to the edges of the channel \nValid Values:\n0 MHz to 120 MHz\n\n<FrequencyEnd>\nStop frequency of the area, relative to the edges of the channel\nValid Values:\n0 MHz to 125 MHz\n\n<Level>\nUpper limit for the area\nValid Values:\n-256 dBm to 256 dBm\n\n<RBW>\nResolution bandwidth to be used for the area\nValid Values:\nK030: 30 kHz\nPC1: 1 % of aggregated channel bandwidth\nM1: 1 MHz\n\nAvailable Repeated Capabilities:\ninstance: i0, i1, i2, i3, i4, i5, i6, i7, i8, i9, i10, i11, i12, i13, i14, i15, i16, i17, i18, i19, i20, i21, i22, i23, i24, i25, i26, i27, i28, i29, i30, i31, i32\r\nArea: a1, a2, a3, a4, a5, a6, a7, a8, a9, a10, a11, a12\r\n\nRemote-control command(s):\nCONFigure:NRSub:MEAS<i>:MEValuation:LIMit:SEMask:AREA<no>:ENDC"}, {"Level"=4, "Class Only"=FALSE, "Identifier"="RSCMWXPNRFR1M_ATTR_MULTI_EVAL_MEAS_LIMIT_SEM_ADDITIONAL_CHANNEL_BW", "Descriptive Name"="Multi Eval Meas Limit SEM Additional Channel BW", "Data Type"=enum."RawString", "Command"="CONF:NRS:MEAS{instance}:MEV:LIM:SEM:AREA{Area}:ADD{Table}:CBAN{Bandwidth}", "Access"=enum."Read/Write", "Range Table"="", "Read Callback"="", "Write Callback"="", "Range Callback"="", "Check Callback"="", "Rngtable Callback"="", "Coerce Callback"="", "Supported Models"="", "Instrument Options"="", "Check Status Callback"="", "Flags"=0, "Help"="Defines additional requirements for the emission mask area number <area> (for NR SA). The activation state, the area borders, an upper limit and the resolution bandwidth must be specified.\nThe emission mask applies to the channel bandwidth <bw>. Several tables of additional requirements are available.\n\nSyntax:\nCONFigure:NRSub:MEAS<i>:MEValuation:LIMit:SEMask:AREA<area>:ADDitional<table>:CBANdwidth<bw> <Enable>, <FrequencyStart>, <FrequencyEnd>, <Level>, <RBW>\n\n<Enable>\nValid Values:\nOFF\nON\n\n<FrequencyStart>\nStart frequency of the area, relative to the edges of the channel bandwidth\nValid Values:\n0 MHz to 105 MHz\n\n<FrequencyEnd>\nStop frequency of the area, relative to the edges of the channel bandwidth\nValid Values:\n0 MHz to 105 MHz\n\n<Level>\nUpper limit for the area\nValid Values:\n-256 dBm to 256 dBm\n\n<RBW>\nResolution bandwidth to be used for the area\nOnly a subset of the values is allowed, depending on <table> and <bw>.\nValid Values:\nK030: 30 kHz\nK100: 100 kHz\nM1: 1 MHz\nPC1: 1 % of channel bandwidth\nPC2: 2 % of channel bandwidth\n\nAvailable Repeated Capabilities:\ninstance: i0, i1, i2, i3, i4, i5, i6, i7, i8, i9, i10, i11, i12, i13, i14, i15, i16, i17, i18, i19, i20, i21, i22, i23, i24, i25, i26, i27, i28, i29, i30, i31, i32\r\nArea: a1, a2, a3, a4, a5, a6, a7, a8, a9, a10, a11, a12\r\nTable: Table1, Table2, Table3, Table4\r\nBandwidth: bw5, bw10, bw15, bw20, bw25, bw30, bw40, bw50, bw60, bw80, bw90, bw100\r\n\nRemote-control command(s):\nCONFigure:NRSub:MEAS<i>:MEValuation:LIMit:SEMask:AREA<area>:ADDitional<table>:CBANdwidth<bw>"}, {"Level"=4, "Class Only"=FALSE, "Identifier"="RSCMWXPNRFR1M_ATTR_MULTI_EVAL_MEAS_LIMIT_SEM_OBW", "Descriptive Name"="Multi Eval Meas Limit SEM OBW", "Data Type"=enum."ViReal64", "Command"="CONF:NRS:MEAS{instance}:MEV:LIM:SEM:OBWL:ENDC", "Access"=enum."Read/Write", "Range Table"="rsCmwxpNrFr1M_rngLimitOBW", "Read Callback"="", "Write Callback"="", "Range Callback"="", "Check Callback"="", "Rngtable Callback"="", "Coerce Callback"="", "Supported Models"="", "Instrument Options"="", "Check Status Callback"="", "Flags"=0, "Help"="Defines an upper limit for the occupied bandwidth, for EN-DC measurements.\n\nAvailable Repeated Capabilities:\ninstance: i0, i1, i2, i3, i4, i5, i6, i7, i8, i9, i10, i11, i12, i13, i14, i15, i16, i17, i18, i19, i20, i21, i22, i23, i24, i25, i26, i27, i28, i29, i30, i31, i32\r\n\nRemote-control command(s):\nCONFigure:NRSub:MEAS<i>:MEValuation:LIMit:SEMask:OBWLimit:ENDC"}, {"Level"=3, "Class Only"=TRUE, "Identifier"="", "Descriptive Name"="Power Dynamics", "Data Type"=enum."ViInt32", "Command"="", "Access"=enum."Read Only", "Range Table"="", "Read Callback"="", "Write Callback"="", "Range Callback"="", "Check Callback"="", "Rngtable Callback"="", "Coerce Callback"="", "Supported Models"="", "Instrument Options"="", "Check Status Callback"="", "Flags"=0, "Help"="Contains attributes for Power Dynamics Limits."}, {"Level"=4, "Class Only"=FALSE, "Identifier"="RSCMWXPNRFR1M_ATTR_MULTI_EVAL_MEAS_LIMIT_POWER_DYNAMICS_ENABLED", "Descriptive Name"="Multi Eval Meas Limit Power Dynamics Enabled", "Data Type"=enum."ViBoolean", "Command"="CONF:NRS:MEAS{instance}:MEV:LIM:PDYN:ENAB", "Access"=enum."Read/Write", "Range Table"="", "Read Callback"="", "Write Callback"="", "Range Callback"="", "Check Callback"="", "Rngtable Callback"="", "Coerce Callback"="", "Supported Models"="", "Instrument Options"="", "Check Status Callback"="", "Flags"=0, "Help"="Enables or disables the limit check for the power dynamics measurement.\n\nAvailable Repeated Capabilities:\ninstance: i0, i1, i2, i3, i4, i5, i6, i7, i8, i9, i10, i11, i12, i13, i14, i15, i16, i17, i18, i19, i20, i21, i22, i23, i24, i25, i26, i27, i28, i29, i30, i31, i32\r\n\nRemote-control command(s):\nCONFigure:NRSub:MEAS<i>:MEValuation:LIMit:PDYNamics:ENABle"}, {"Level"=4, "Class Only"=FALSE, "Identifier"="RSCMWXPNRFR1M_ATTR_MULTI_EVAL_MEAS_LIMIT_POWER_DYNAMICS_OFF_POWER", "Descriptive Name"="Multi Eval Meas Limit Power Dynamics OFF Power", "Data Type"=enum."ViReal64", "Command"="CONF:NRS:MEAS{instance}:MEV:LIM:PDYN:OFFP", "Access"=enum."Read/Write", "Range Table"="rsCmwxpNrFr1M_rngPDYNOFFPower", "Read Callback"="", "Write Callback"="", "Range Callback"="", "Check Callback"="", "Rngtable Callback"="", "Coerce Callback"="", "Supported Models"="", "Instrument Options"="", "Check Status Callback"="", "Flags"=0, "Help"="Defines an upper limit for the OFF power determined with the power dynamics measurement.\n\nAvailable Repeated Capabilities:\ninstance: i0, i1, i2, i3, i4, i5, i6, i7, i8, i9, i10, i11, i12, i13, i14, i15, i16, i17, i18, i19, i20, i21, i22, i23, i24, i25, i26, i27, i28, i29, i30, i31, i32\r\n\nRemote-control 
